vi "Global_CMD Data.vi"() -> ()   [LabVIEW 2017, in "TemplateActuator.lvlib"]
uses:
  TemplateActuator.lvlib
  Cluster_CMD to SM Data.ctl
  ENUM_SM Cmd Select.ctl
panel:
  in  "CMD_Actuator Data":T1
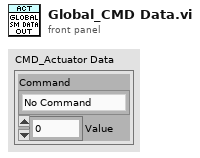
[diagram p1: front panel]
types:
  T1 = typedef "TemplateActuator.lvlib/Cluster_CMD to SM Data.ctl" = cluster{"Command":T2, "Value":dbl}
  T2 = typedef "TemplateActuator.lvlib/ENUM_SM Cmd Select.ctl" = enum16{"No Command", "Stop", "Go"}
diagram:
